vi "SV Peak Hold Spectra (Complex).vi"(0 "complex spectra":T7(array[cluster]) {"spectrum info"."x-axis units" items=["Time (s)"=0, "Frequency-CB (Hz)"=1, "Frequency-CPB (Hz)"=1248, "Frequency-Arbitrary (Hz)"=2357, "Quefrency (s)"=2, "Revolutions (rev)"=3, "Order"=4, "Speed (RPM)"=11, "Speed (rad/s)"=21, "Index"=65535]; "spectrum info"."weighting filter" items=["Linear", "A-weighting", "B-weighting", "C-weighting", "ITU-R 468-4", "Dolby", "CCITT", "C-message", "Wb", "Wc", "Wd", "We", "Wf", "Wh", "Wj", "Wk", "Wm", "AES17 20 kHz lowpass", "AES17 40 kHz lowpass", "AES17 20 kHz highpass", "AES17 40 kHz highpass"]; "spectrum info"."dB reference [EU]" format="%.2f"; "spectrum info"."engineering units" items=["custom..."=0, "V"=1, "A"=21, "C"=30, "pC"=31, "s"=32, "-"=29, "Pa"=2, "N"=20, "g"=3, "m/s^2"=4, "m/s"=5, "m"=6, "mm/s"=12, "mm"=13, "micron/s"=14, "micron"=15, "in/s^2"=7, "in/s"=8, "in"=9, "mil/s"=10, "mil"=11, "rad/s^2"=16, "rad/s"=17, "rad"=18, "deg/s^2"=26, "deg/s"=27, "deg"=28, "RPM"=22, "cycle/s^2"=23, "Hz"=24, "cycle"=25, "strain"=19]; "spectrum info"."spectral info"."window" items=["None "=0, "Hanning"=1, "Hamming"=2, "Blackman-Harris"=3, "Exact Blackman"=4, "Blackman"=5, "Flat Top"=6, "4 Term B-Harris "=7, "7 Term B-Harris"=8, "Low Sidelobe"=9, "Force - Exponential"=10, "Gaussian"=62]; "complex spectrum response"."complex spectrum" format="%.2f"; "complex spectrum response"."df" format="%.2f"; "complex spectrum response"."f0" format="%.2f"}, 5 "error in (no error)":errorcluster) -> (13 "averages completed":dbl, 14 "peak hold magnitude spectrum":cluster{"f0":dbl, "df":dbl, "magnitude":dbl[]} {"magnitude" format="%.2p"; "df" format="%.2p"; "f0" format="%.2p"}, 18 "spectrum info":T1={"channel name"="", "description"="", "x-axis units"=0, "spectral info"={"spectrum type"=enum."Power [Magnitude^2]", "linear/dB"=enum."linear", "window"=0, "window size"=0, "FFT size"=0}, "engineering units"=1, "custom label"="", "dB reference [EU]"=0.0, "peak units"=enum."rms", "weighting filter"=0, "spectral density?"=FALSE, "unit label"="", "spectrum skewed?"=FALSE, "complimentary spectrum units"=enum."none"} {"x-axis units" items=["Time (s)"=0, "Frequency-CB (Hz)"=1, "Frequency-CPB (Hz)"=1248, "Frequency-Arbitrary (Hz)"=2357, "Quefrency (s)"=2, "Revolutions (rev)"=3, "Order"=4, "Speed (RPM)"=11, "Speed (rad/s)"=21, "Index"=65535]; "weighting filter" items=["Linear", "A-weighting", "B-weighting", "C-weighting", "ITU-R 468-4", "Dolby", "CCITT", "C-message", "Wb", "Wc", "Wd", "We", "Wf", "Wh", "Wj", "Wk", "Wm", "AES17 20 kHz lowpass", "AES17 40 kHz lowpass", "AES17 20 kHz highpass", "AES17 40 kHz highpass"]; "dB reference [EU]" format="%.2f"; "engineering units" items=["custom..."=0, "V"=1, "A"=21, "C"=30, "pC"=31, "s"=32, "-"=29, "Pa"=2, "N"=20, "g"=3, "m/s^2"=4, "m/s"=5, "m"=6, "mm/s"=12, "mm"=13, "micron/s"=14, "micron"=15, "in/s^2"=7, "in/s"=8, "in"=9, "mil/s"=10, "mil"=11, "rad/s^2"=16, "rad/s"=17, "rad"=18, "deg/s^2"=26, "deg/s"=27, "deg"=28, "RPM"=22, "cycle/s^2"=23, "Hz"=24, "cycle"=25, "strain"=19]; "spectral info"."window" items=["None "=0, "Hanning"=1, "Hamming"=2, "Blackman-Harris"=3, "Exact Blackman"=4, "Blackman"=5, "Flat Top"=6, "4 Term B-Harris "=7, "7 Term B-Harris"=8, "Low Sidelobe"=9, "Force - Exponential"=10, "Gaussian"=62]}, 19 "error out":errorcluster)   [LabVIEW 2017]
doc: "Computes the linear RMS-averaged power spectrum of <B>scaled signal [EU]</B> in a linear scale. Use the power spectrum to quantify signal components as a function of frequency. Use this VI on embedded targets that have limited computational resources. Wire data to the <B>scaled signal [EU]</B> input to determine the polymorphic instance to use or manually select the instance."
uses:
  <vilib>/addons/_NISVFA/_Shared subVIs/Controls/svc_Spectrum Info.ctl
  <vilib>/addons/_NISVFA/_Shared subVIs/Controls/svc_X-Axis Units.ctl
  <vilib>/addons/_NISVFA/_Shared subVIs/Controls/svc_Spectrum Type.ctl
  <vilib>/addons/_NISVFA/_Shared subVIs/Controls/svc_Engineering Units Text Ring.ctl
  <vilib>/addons/_NISVFA/_Shared subVIs/Controls/svc_Weighting Filter Text Ring.ctl
  <vilib>/addons/_NISVFA/_Shared subVIs/Controls/svc_Complimentary Spectrum Units.ctl
  <vilib>/addons/_NISVFA/_Shared subVIs/Common/svc_Get Weighting Enum and Labels.vi
  <vilib>/addons/_NISVFA/_Shared subVIs/Common/svc_Unit Label Lexical Class.vi
  <vilib>/addons/_NISVFA/_Shared subVIs/Common/svc_Engineering Units to Unit Label.vi
  <vilib>/addons/_NISVFA/_Shared subVIs/Common/svc_Format Value (DBL).vi
  <vilib>/addons/_NISVFA/_Spectrum Processing/SVFA Unit Conversion (Complex) (1 Ch).vi
panel:
  out "unit label":string
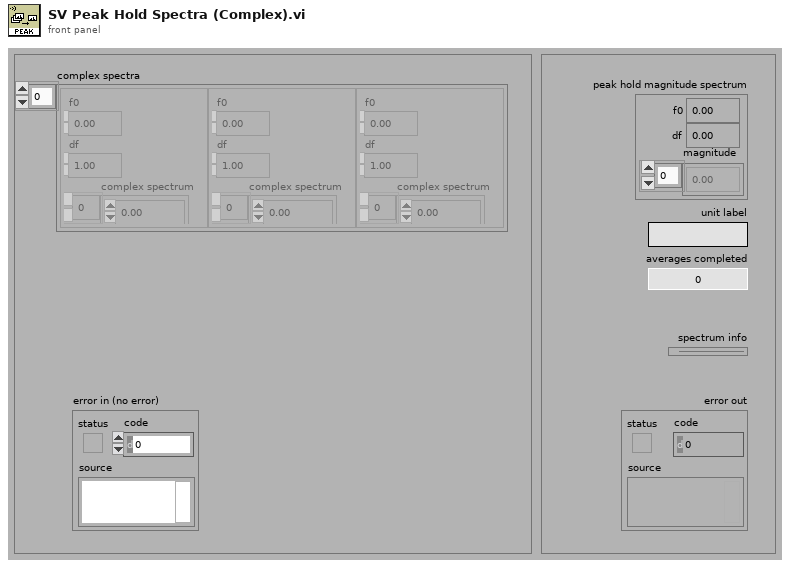
[diagram p1: front panel]
types:
  T1 = typedef "svc_Spectrum Info.ctl" = cluster{"channel name":string, "description":string, "x-axis units":T2, "spectral info":cluster{"spectrum type":T3, "linear/dB":enum16{"linear", "dB"}, "window":u16, "window size":i32, "FFT size":i32}, "engineering units":T4, "custom label":string, "dB reference [EU]":dbl, "peak units":enum16{"rms", "peak", "peak-peak"}, "weighting filter":T5, "spectral density?":bool, "unit label":string, "spectrum skewed?":bool, "complimentary spectrum units":T6}
  T2 = typedef "svc_X-Axis Units.ctl" = u16
  T3 = typedef "svc_Spectrum Type.ctl" = enum16{"FFT Spectrum [complex]", "Amplitude [Magnitude]", "Power [Magnitude^2]", "Cross Spectrum [complex]", "Frequency Response [Complex]"}
  T4 = typedef "svc_Engineering Units Text Ring.ctl" = u16
  T5 = typedef "svc_Weighting Filter Text Ring.ctl" = u16
  T6 = typedef "svc_Complimentary Spectrum Units.ctl" = enum16{"none", "radians", "degrees", "cycles", "imaginary"}
  T7 = cluster{"complex spectrum response":cluster{"f0":dbl, "df":dbl, "complex spectrum":cdb[]}, "spectrum info":T1}[]
  T8 = cluster{"linear/dB":enum16{"no change", "linear", "dB"}, "dB reference (0: no change)":dbl, "power/magnitude":enum16{"no change", "power", "magnitude"}, "view":enum16{"no change", "rms", "peak", "peak-peak"}}
  T9 = enum16{"Restart processing", "Continue processing", "Skip processing"}
  T10 = cluster{"complex spectrum response":cluster{"f0":dbl, "df":dbl, "complex spectrum":cdb[]}, "spectrum info":T1}
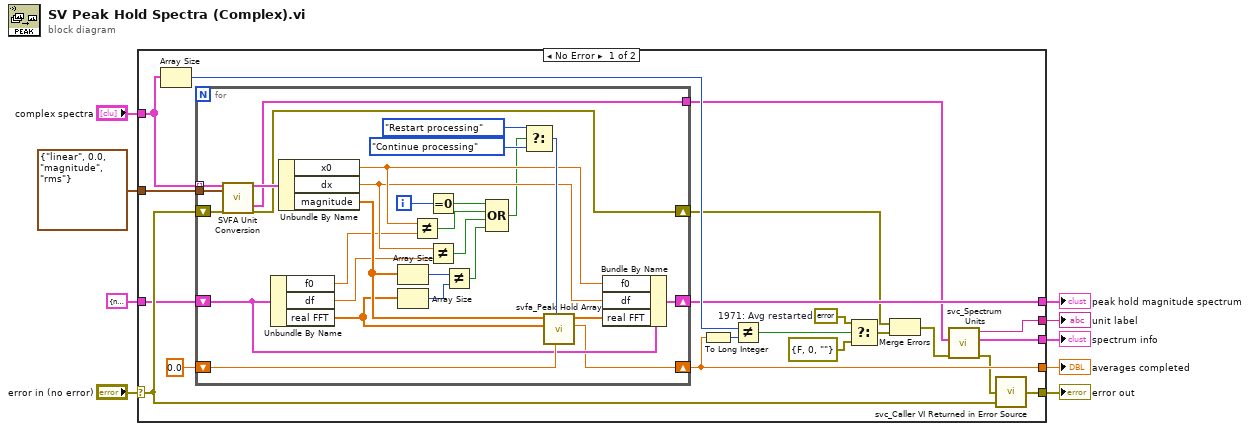
[diagram p0: block diagram]
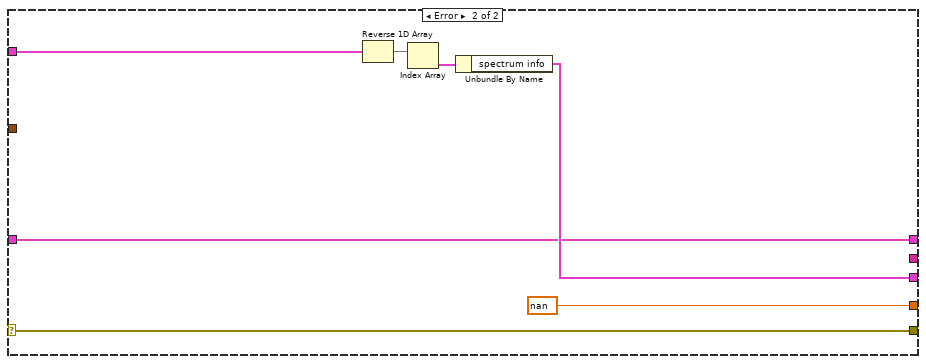
[diagram p2: hidden frame]
diagram:
  n1 = case shown="No Error" "error in (no error)" {
    selector: "error in (no error)" -> [w20 w63]
    tunnel: [w19 w58] -> w6
    tunnel: "complex spectra" -> [w21 w62]
    tunnel: [w28 nan ("Numeric")] -> w3
    tunnel: [w22 w63] -> w2
    tunnel: [w15 w59] -> w5
    tunnel: T8 {"linear/dB"=enum."linear", "dB reference (0: no change)"=0.0, "power/magnitude"=enum."magnitude", "view"=enum."rms"} ("desired scaling") -> [w16 _]
    tunnel: [w11 _] -> w4
    tunnel: cluster{"f0":dbl, "df":dbl, "real FFT":dbl[]} {"f0"=nan, "df"=nan, "real FFT"=[]} ("previous avg real spectrum") -> [w10 w58]
    frame No Error {
      w25 = errorcluster {"status"=FALSE, "code"=1971, "source"="<append>\nAveraging restarted due to change in f0, df, or spectrum size within complex spectra input."}  # 1971: Avg restarted
      n2 = Array Size(array=w21) -> (size(s)=w27:i32)
      n3 = for {
        tunnel: w21 -> [w30] mode=indexing
        shift-right: [w38] -> w28
        shift-left: 0.0 ("Numeric") -> [w47]
        shift-right: [w40] -> w19
        shift-left: w10 -> [w44]
        tunnel: w16 -> [w34]
        shift-right: [w32] -> w18
        shift-left: w20 -> [w33]
        tunnel: [w31] -> w14
        i -> [w45]
        n4 = call-poly <vilib>:"SVFA Unit Conversion.vi"("complex spectrum"=w30, "desired scaling"=w34, "error in (no error)"=w33) -> ("converted spectrum"=w35:cluster{"x0":dbl, "dx":dbl, "magnitude":dbl[]}, "spectrum info out"=w31:T1, "error out"=w32:errorcluster)  [unwired: 11 in, 3 out]
        n5 = Unbundle By Name(w44) -> ("f0"=w37:dbl, "df"=w36:dbl, "real FFT"=w48:dbl[])
        n6 = Unbundle By Name(w35) -> ("x0"=w42:dbl, "dx"=w41:dbl, "magnitude"=w57:dbl[])
        n7 = Array Size(array=w57) -> (size(s)=w56:i32)
        n8 = Array Size(array=w48) -> (size(s)=w55:i32)
        n9 = Not Equal?(x=w42, y=w37) -> (x != y?=w54:bool)
        n10 = Equal To 0?(x=w45) -> (x = 0?=w46:bool)
        n11 = Not Equal?(x=w41, y=w36) -> (x != y?=w50:bool)
        n12 = Not Equal?(x=w56, y=w55) -> (x != y?=w53:bool)
        n13 = Compound Arithmetic op=OR(w46, w54, w50, w53) -> (w39:bool)
        n14 = Select(t=T9."Restart processing", s=w39, f=T9."Continue processing" ("processing control")) -> (s? t:f=w49:T9)
        n15 = call <vilib>:"svfa_Peak Hold Array.vi"("averages completed in"=w47, "processing control"=w49, "previous peak array"=w48, "array"=w57) -> ("averages completed out"=w38:dbl, "peak array"=w43:dbl[])  [unwired: 5 in, 1 out]
        n16 = Bundle By Name(cluster=w44, "f0"=w42, "df"=w41, "real FFT"=w43) -> (w40:cluster{"f0":dbl, "df":dbl, "real FFT":dbl[]})
      }
      n17 = To Long Integer(number=w28) -> (32bit integer=w26:i32)
      n18 = Not Equal?(x=w27, y=w26) -> (x != y?=w23:bool)
      n19 = Select(t=w25, s=w23, f=errorcluster {"status"=FALSE, "code"=0, "source"=""}) -> (s? t:f=w17:errorcluster)
      n20 = Merge Errors(w18, w17) -> (w13:errorcluster)
      n21 = call <vilib>:"svc_Spectrum Units.vi"("error in (no error)"=w13, "spectrum info in"=w14) -> ("error out"=w12:errorcluster, "spectrum info out"=w15:T1, "unit label"=w11:string)  [unwired: 2 in, 1 out]
      n22 = call <vilib>:"svc_Caller VI Returned in Error Source.vi"("warning input to caller"=w20, "error in (no error)"=w12) -> ("error out"=w22:errorcluster)  [unwired: 3 in]
    }
    frame Error {
      n23 = Reverse 1D Array(array=w62) -> (reversed array=w61:T7)
      n24 = Index Array(array=w61) -> (element=w60:T10)  [unwired: 1 in]
      n25 = Unbundle By Name(w60) -> ("spectrum info"=w59:T1)
    }
  }
  "peak hold magnitude spectrum" <- w6
  "averages completed" <- w3
  "error out" <- w2
  "spectrum info" <- w5
  "unit label" <- w4
